vi "TabJoinLines.vi"(11 "Array":string[](array[string])) -> (3 "String":string)   [LabVIEW 2017]
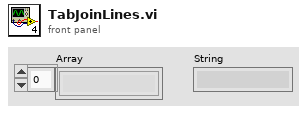
[diagram p1: front panel]
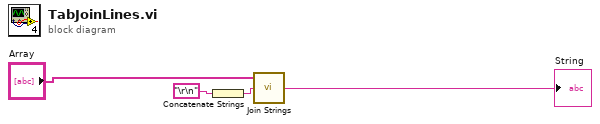
[diagram p0: block diagram]
diagram:
  n1 = Concatenate Strings("\r\n") -> (w3:string)
  n2 = call <vilib>:"Join Strings.vi"("Separator (,)"=w3, "Strings In"="Array") -> ("String"=→"String":string)  [unwired: 1 in]
